vi "_Write File Header.vi"(4 "error in (no error)":errorcluster, 5 "Sample Info":string[](array[string]), 6 "AcqMethod":T1[](array[typedef]) {"ScanType" format="%#.6g"; "Mass Range"."Res" items=["High/High", "Medium/Medium", "Low/Low", "High/Medium", "High/Low", "Medium/High", "Medium/Low", "Low/High", "Low/Medium"]}, 7 "File Refnum In":refnum<file>) -> (0 "error out":errorcluster, 1 "offset":i64, 3 "File Refnum Out":refnum<file>)   [LabVIEW 2015]
uses:
  Type/_XML Expt.ctl
  Type/_XML Lens.ctl
  Type/_Mass Range Property.ctl
  Type/_Mass Range Parameters.ctl
  Type/_RT Res Type.ctl
  Configuration/_Global Configuration.vi
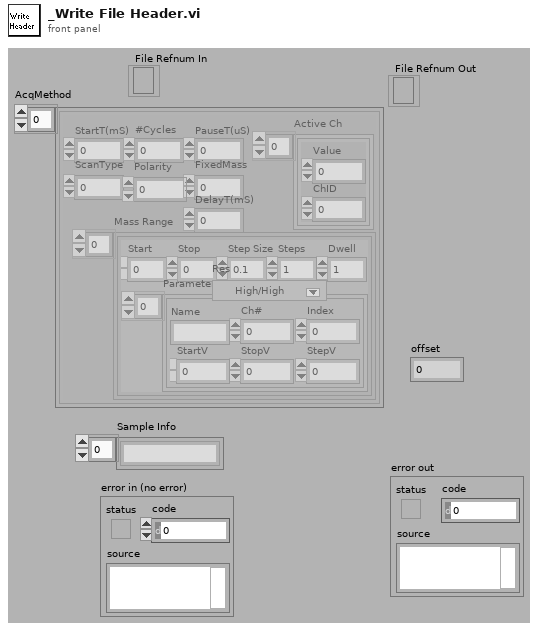
[diagram p1: front panel]
types:
  T1 = typedef "_XML Expt.ctl" = cluster{"StartT(mS)":i32, "#Cycles":i32, "PauseT(uS)":i32, "ScanType":i32, "Polarity":u8, "FixedMass":dbl, "DelayT(mS)":i32, "Active Ch":T2[], "Mass Range":T3[]}
  T2 = typedef "_XML Lens.ctl" = cluster{"Value":dbl, "ChID":u8}
  T3 = typedef "_Mass Range Property.ctl" = cluster{"Start":dbl, "Stop":dbl, "Step Size":dbl, "Steps":i32, "Dwell":dbl, "Parameters":T4[], "Res":T5}
  T4 = typedef "_Mass Range Parameters.ctl" = cluster{"Name":string, "Ch#":u8, "StartV":dbl, "StopV":dbl, "StepV":dbl, "Index":u8}
  T5 = typedef "_RT Res Type.ctl" = u16
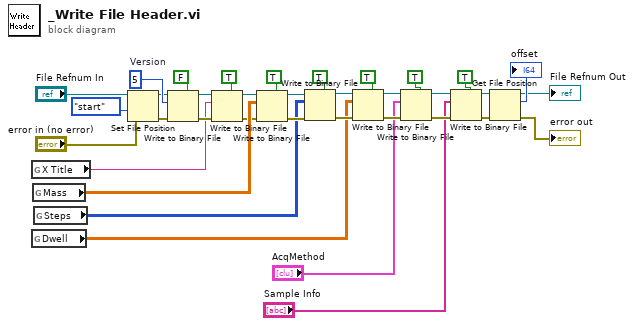
[diagram p0: block diagram]
diagram:
  w34 = 5  # Version
  n1 = global read "_Global Configuration.vi" "X Title"() -> (w14:string)
  n2 = global read "_Global Configuration.vi" "Dwell"() -> (w8:dbl[][])
  n3 = global read "_Global Configuration.vi" "Mass"() -> (w31:dbl[][])
  n4 = global read "_Global Configuration.vi" "Steps"() -> (w30:i32[][])
  n5 = Set File Position(refnum="File Refnum In", from (0:start)=enum16{"start", "end", "current"}."start" ("pos mode (0:2)"), error in="error in (no error)") -> (refnum out=w28:refnum<file>, error out=w27:errorcluster)  [unwired: 1 in]
  n6 = Write to Binary File(file (use dialog)=w28, data=w34, error in=w27, 5:FALSE ("prepend array or string size? (T)")) -> (refnum out=w17:refnum<file>, error out=w18:errorcluster)  [unwired: 3 out]
  n7 = Write to Binary File(file (use dialog)=w17, data=w14, error in=w18, 5:TRUE ("prepend array or string size? (T)")) -> (refnum out=w15:refnum<file>, error out=w16:errorcluster)  [unwired: 3 out]
  n8 = Write to Binary File(file (use dialog)=w15, data=w31, error in=w16, 5:TRUE ("prepend array or string size? (T)")) -> (refnum out=w33:refnum<file>, error out=w32:errorcluster)  [unwired: 3 out]
  n9 = Write to Binary File(file (use dialog)=w33, data=w30, error in=w32, 5:TRUE ("prepend array or string size? (T)")) -> (refnum out=w11:refnum<file>, error out=w10:errorcluster)  [unwired: 3 out]
  n10 = Write to Binary File(file (use dialog)=w11, data=w8, error in=w10, 5:TRUE ("prepend array or string size? (T)")) -> (refnum out=w9:refnum<file>, error out=w12:errorcluster)  [unwired: 3 out]
  n11 = Write to Binary File(file (use dialog)=w9, data="AcqMethod", error in=w12, 5:TRUE ("prepend array or string size? (T)")) -> (refnum out=w4:refnum<file>, error out=w5:errorcluster)  [unwired: 3 out]
  n12 = Write to Binary File(file (use dialog)=w4, data="Sample Info", error in=w5, 5:TRUE ("prepend array or string size? (T)")) -> (refnum out=w3:refnum<file>, error out=w2:errorcluster)  [unwired: 3 out]
  n13 = Get File Position(4:w2, 7:w3) -> (0:→"error out":errorcluster, 2:→"offset":i64, 3:→"File Refnum Out":refnum<file>)
